vi "型号到特定类(数表)转换.vi"(8 "error in (no error)":errorcluster caption="错误输入（无错误）", 11 "型号":string) -> (0 "错误输出":errorcluster, 3 "DMM":refnum<class "数字多用表接口.lvclass">)   [LabVIEW 2020]
uses:
  <vilib>/Utility/LVLibp/NI_PackedLibraryUtility.lvlib
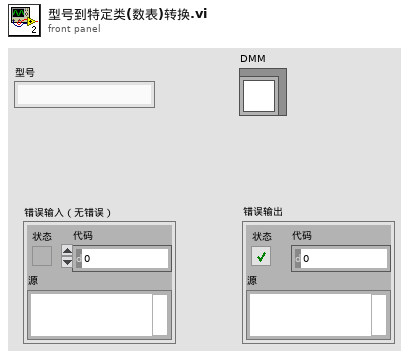
[diagram p1: front panel]
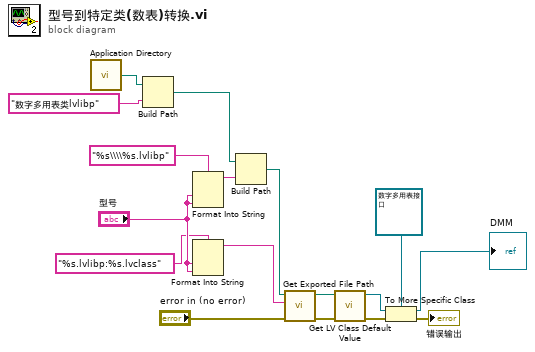
[diagram p0: block diagram]
diagram:
  n1 = call <vilib>:"Application Directory.vi"() -> ("Application Directory"=w3:path)
  n2 = Build Path(base path=w3, name or relative path="数字多用表类lvlibp" ("名称或相对路径")) -> (appended path=w2:path)
  n3 = Format Into String(format string="%s\\\\%s.lvlibp" ("名称或相对路径"), "型号", "型号") -> (resulting string=w11:string)  [unwired: 2 in, 1 out]
  n4 = Format Into String(format string="%s.lvlibp:%s.lvclass" ("名称或相对路径"), "型号", "型号") -> (resulting string=w13:string)  [unwired: 2 in, 1 out]
  n5 = Build Path(base path=w2, name or relative path=w11) -> (appended path=w12:path)
  n6 = call <vilib>:"Get Exported File Path.vi"("error in (no error)"="error in (no error)", "qualified name"=w13, "packed library path"=w12) -> ("error out"=w15:errorcluster, "path"=w14:path)  [unwired: 7 in]
  n7 = call <vilib>:"Get LV Class Default Value.vi"("error in (no error)"=w15, "class path"=w14) -> ("error out"=w17:errorcluster, "object"=w16:refnum<class>)  [unwired: 8 in]
  n8 = To More Specific Class(target class=refnum<class "数字多用表接口.lvclass"> refnum ("数字多用表接口.lvlibp:数字多用表接口.lvclass"), reference=w16, error in=w17) -> (specific class reference=→"DMM":refnum<class "数字多用表接口.lvclass">, error out=→"错误输出":errorcluster)
